vi "gbtpFitWithEstimate.vi"(0 "X":dbl[](array[numeric]), 2 "terminationPars":cluster{"max iteration":i32, "tolerance":dbl}={"max iteration"=200, "tolerance"=1e-08}, 3 "imageArray":u16[](array[numeric])) -> (4 "errorOut":errorcluster, 5 "fitPars":dbl[](array[numeric]) format="%#_4g", 6 "fitCovariance":T1 format="%#_4g", 8 "fitY":dbl[](array[numeric]))   [LabVIEW 2021]
uses:
  <vilib>/Analysis/Matrix/Datatypes/RealMatrix.ctl
  <vilib>/gmath/NumericalOptimization/Nonlinear Curve Fit LM.vi
  <vilib>/gmath/NI_Gmath.lvlib
  <vilib>/Analysis/Matrix/NI_Matrix.lvlib
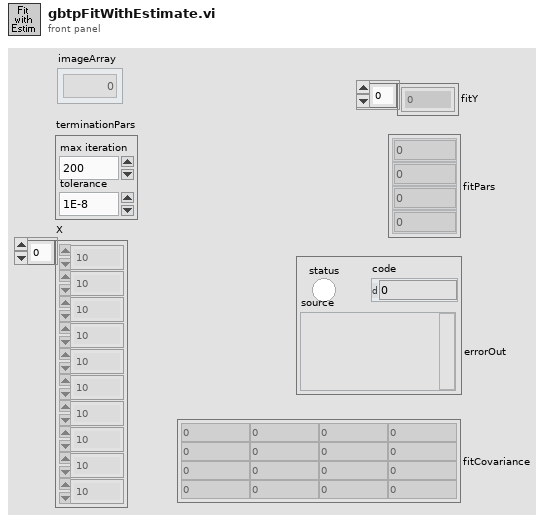
[diagram p1: front panel]
types:
  T1 = typedef "NI_Matrix.lvlib/RealMatrix.ctl" = dbl[][]
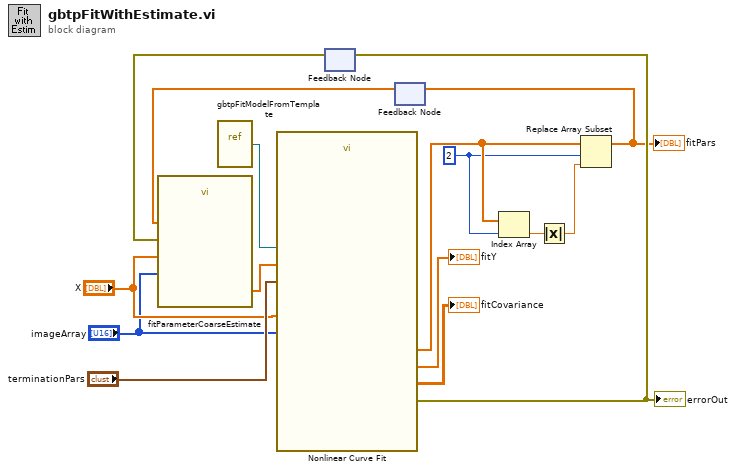
[diagram p0: block diagram]
diagram:
  w4 = 2 ("index")
  n1 = vi-ref "gbtpFitModelFromTemplate.vi"() -> (w14:refnum<vi>)
  n2 = feedback #1() -> (w8:errorcluster)  [unwired: 1 in]
  n3 = feedback #2() -> (w9:dbl[])  [unwired: 1 in]
  n4 = call "fitParameterCoarseEstimate.vi"("erroIn"=w8, "Y"="imageArray", "X"="X", "previousPars"=w9) -> ("pars"=w15:dbl[])
  n5 = call-poly <vilib>:"Nonlinear Curve Fit.vi"("Y"="imageArray", "f(x,a)"=w14, "X"="X", "initial parameters"=w15, "termination"="terminationPars") -> ("best nonlinear fit"=→"fitY":dbl[], "best fit parameters"=w5:dbl[], "covariance"=→"fitCovariance":T1, "error out"=w7:errorcluster)  [unwired: 5 in, 2 out]
  "errorOut" <- w7
  n6 = feedback-in #1(w7) -> ()
  n7 = Index Array(array=w5, index=w4) -> (element=w3:dbl)
  n8 = Absolute Value(x=w3) -> (abs(x)=w2:dbl)
  n9 = Replace Array Subset(array=w5, new element=w2, index=w4) -> (w1:dbl[])
  "fitPars" <- w1
  n10 = feedback-in #2(w1) -> ()
